vi "RT Init.vi"(6 "Device Outputs FIFO":refnum<k33>, 8 "error in":errorcluster, 11 "Device Ref":T13=18446744073709551615 format="%.0x") -> (0 "error out":errorcluster, 3 "RT Data":T1={"Timekeeper hdl"="", "clkDisc session"=variant, "Compiled Data"={"SyncMod?"=FALSE, "SyncMod"="", "ConnectionSettings"={"Mode"=enum."Generate sample clock", "pxitrig"=FALSE, "pfi0"=FALSE, "pfi1"=FALSE, "pfi2"=FALSE, "External Pin"=enum."PFI0", "Routes"=[]}, "TimeKeeper"="", "ScanOffset(%)"=0.0, "StartDelay(s)"=0, "Time Ref Settings"={"Time Reference"=enum."GPS", "Priority 1"=0, "Priority 2"=0, "IRIG type"=enum."IRIGB AM", "Terminal"="", "PPSSetTime"=FALSE, "Start Time"=timestamp(0 s since 1904-01-01)}, "FIFO Locations"={"BoardTime"=[], "Status"=[]}}, "OutputsData"=[], "OutputsFIFO"=refnum, "Scan Period"=0, "Timekeeper type"=enum."6683", "SyncMod type"=enum."6683", "SyncMod hdl"=""} {"Compiled Data"."Time Ref Settings"."Priority 2" min=0 max=255; "Compiled Data"."Time Ref Settings"."Priority 1" min=0 max=255}, 4 "Name":string)   [LabVIEW 2015, in "Chassis TimeSync Engine.lvlib"]
uses:
  Chassis TimeSync Engine.lvlib
  <vilib>/NI Veristand/Custom Device API/Custom Device Item Ref.ctl
  RT Data Cluster.ctl
  mdevClkDisc.llb/_clkDisc_session.ctl
  Shared/Compiled Data.ctl
  Shared/Connection Settings.ctl
  Shared/Mode.ctl
  Shared/External Pin.ctl
  Shared/Routes.ctl
  Shared/Route.ctl
  Shared/Time Ref Settings.ctl
  Shared/Time Reference.ctl
  Shared/IRIG Type.ctl
  timekeeper type.ctl
  <instrlib>/niSync/niSync.llb/niSync Initialize (Default).vi
  <vilib>/NI Veristand/Custom Device API/Get Item Property (Variant).vi
  Shared/Constants.vi
  <vilib>/NI Veristand/Custom Device API/Custom Device API.lvlib
  Shared/Chassis TimeSync Shared.lvlib
  <vilib>/NI Veristand/Custom Device Tools/Custom Device Utility Library/Custom Device Utility Library.lvlib
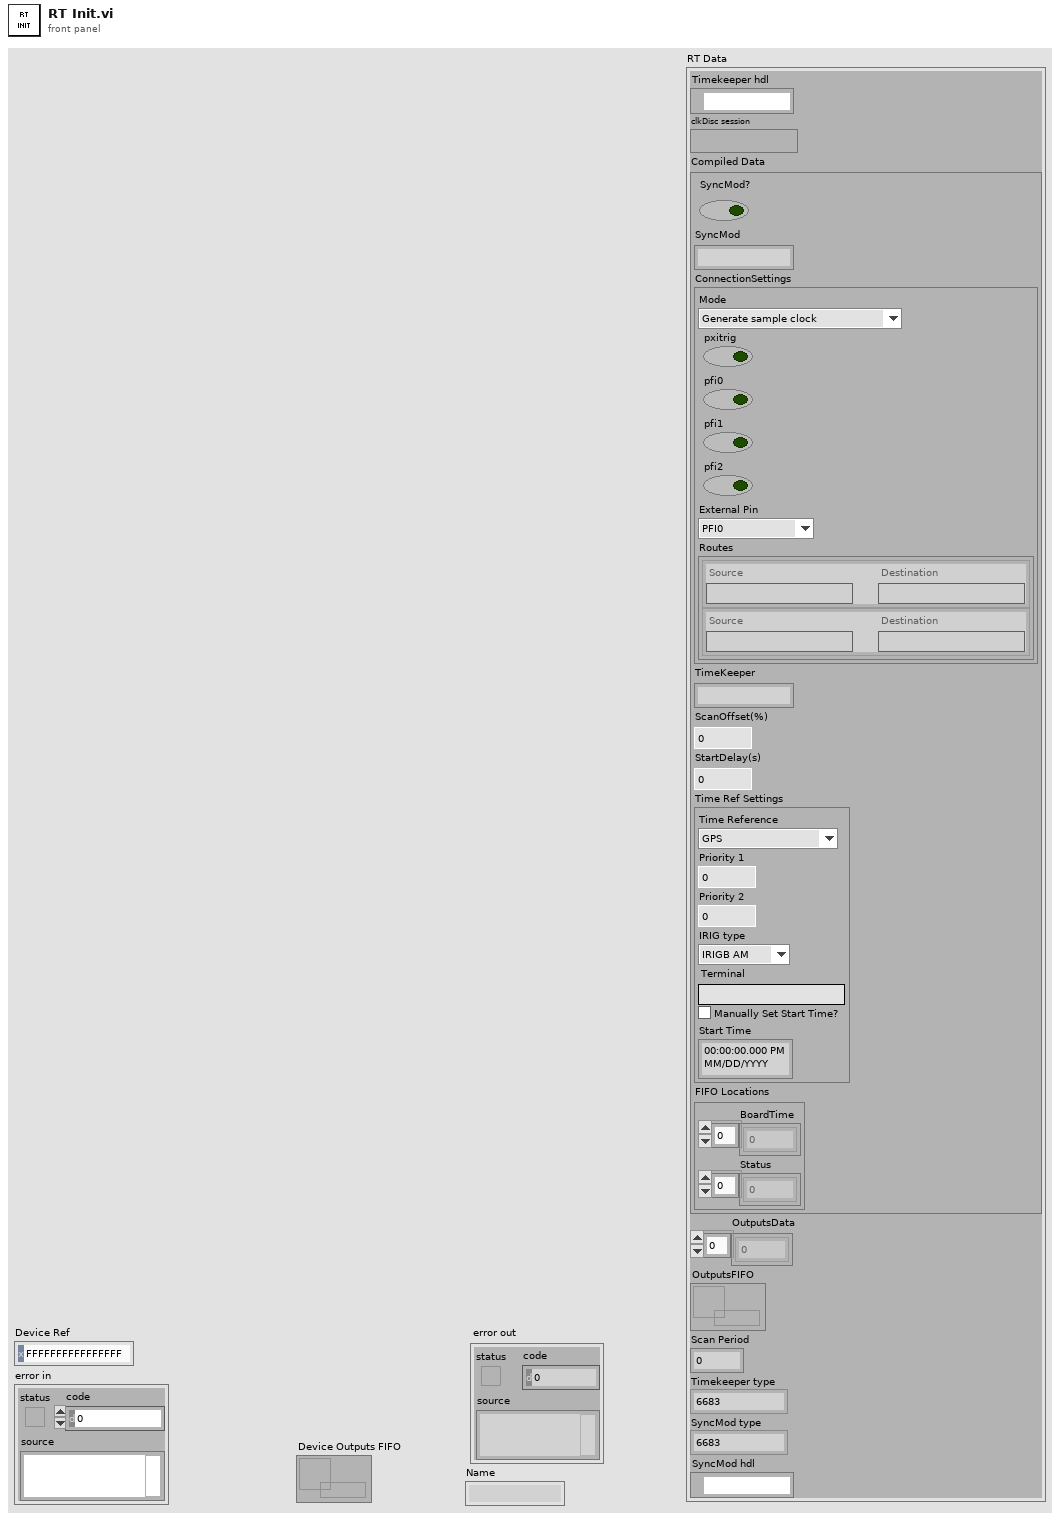
[diagram p1: front panel]
types:
  T1 = typedef "Chassis TimeSync Engine.lvlib/RT Data Cluster.ctl" = cluster{"Timekeeper hdl":refnum<k15>, "clkDisc session":T2, "Compiled Data":T3, "OutputsData":dbl[], "OutputsFIFO":refnum<k33>, "Scan Period":u32, "Timekeeper type":T12, "SyncMod type":T12, "SyncMod hdl":refnum<k15>}
  T2 = typedef "_clkDisc_session.ctl" = variant
  T3 = typedef "Chassis TimeSync Shared.lvlib/Compiled Data.ctl" = cluster{"SyncMod?":bool, "SyncMod":string, "ConnectionSettings":T4, "TimeKeeper":string, "ScanOffset(%)":dbl, "StartDelay(s)":u16, "Time Ref Settings":T9, "FIFO Locations":cluster{"BoardTime":i32[], "Status":i32[]}}
  T4 = typedef "Chassis TimeSync Shared.lvlib/Connection Settings.ctl" = cluster{"Mode":T5, "pxitrig":bool, "pfi0":bool, "pfi1":bool, "pfi2":bool, "External Pin":T6, "Routes":T7}
  T5 = typedef "Chassis TimeSync Shared.lvlib/Mode.ctl" = enum16{"Generate sample clock", "Route sample clock out of chassis", "Route sample clock into chassis", "Custom routes"}
  T6 = typedef "Chassis TimeSync Shared.lvlib/External Pin.ctl" = enum16{"PFI0", "PFI1", "PFI2"}
  T7 = typedef "Chassis TimeSync Shared.lvlib/Routes.ctl" = T8[]
  T8 = typedef "Chassis TimeSync Shared.lvlib/Route.ctl" = cluster{"Source":string, "Destination":string}
  T9 = typedef "Chassis TimeSync Shared.lvlib/Time Ref Settings.ctl" = cluster{"Time Reference":T10, "Priority 1":i32, "Priority 2":i32, "IRIG type":T11, "Terminal":string, "PPSSetTime":bool, "Start Time":timestamp}
  T10 = typedef "Chassis TimeSync Shared.lvlib/Time Reference.ctl" = enum16{"GPS", "IRIG", "PPS", "1588 Ordinary Clock", "PXI Chassis Clock", "Free Running (Internal)"}
  T11 = typedef "Chassis TimeSync Shared.lvlib/IRIG Type.ctl" = enum16{"IRIGB DC", "IRIGB AM"}
  T12 = typedef "Chassis TimeSync Engine.lvlib/timekeeper type.ctl" = enum16{"6683", "6683H", "6682", "6682H", "non-timekeeper", "timekeeper"}
  T13 = typedef "Custom Device API.lvlib/Custom Device Item Ref.ctl" = u64
  T14 = typedef "Custom Device API.lvlib/Custom Device Item Info.ctl" = cluster{"Name":string, "Is Channel":bool, "GUID":string, "Is Waveform":bool}
  T15 = typedef "Custom Device API.lvlib/Custom Device Channel.ctl" = cluster{"Type":T16, "Units":string, "Default Value":dbl, "Faultable":bool, "Scalable":bool}
  T16 = typedef "Custom Device API.lvlib/Custom Device Channel Type.ctl" = enum16{"Input", "Output"}
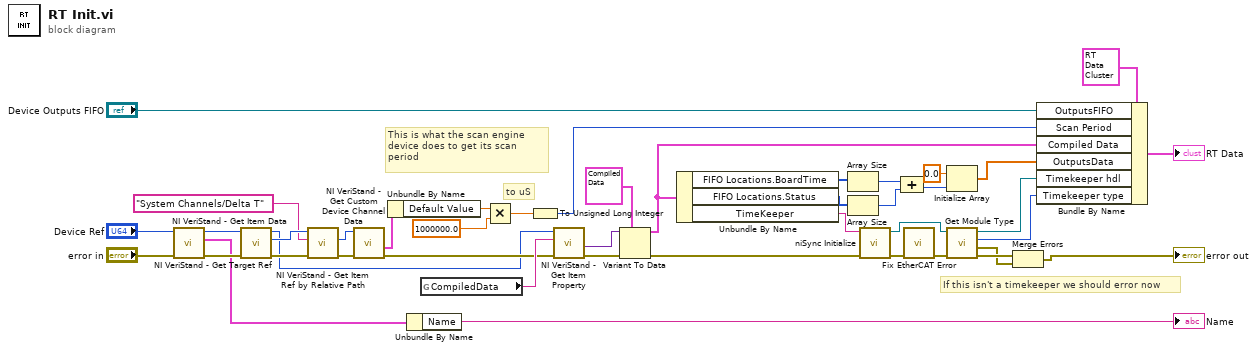
[diagram p0: block diagram]
diagram:
  # "If this isn't a timekeeper we should error now"
  # "This is what the scan engine device does to get its scan period"
  # "to uS"
  n1 = call <vilib>:"NI VeriStand - Get Item Data.vi"("error in (no error)"="error in", "Item Ref in"="Device Ref") -> ("error out"=w13:errorcluster, "Item Info"=w10:T14, "Item Ref out"=w11:T13)  [unwired: 6 in, 1 out]
  n2 = call <vilib>:"NI VeriStand - Get Target Ref.vi"("error in"=w13, "Item Ref in"=w11) -> ("error out"=w21:errorcluster, "Target Ref"=w22:T13, "Item Ref out"=w14:T13)  [unwired: 6 in, 1 out]
  n3 = call <vilib>:"NI VeriStand - Get Item Ref by Relative Path.vi"("error in"=w21, "Relative Item Path"="System Channels/Delta T", "Section Ref in"=w22) -> ("error out"=w18:errorcluster, "Item Ref"=w19:T13)  [unwired: 5 in, 2 out]
  n4 = call <vilib>:"NI VeriStand - Get Custom Device Channel Data.vi"("error in (no error)"=w18, "Channel Ref in"=w19) -> ("error out"=w15:errorcluster, "Channel"=w17:T15)  [unwired: 4 in, 4 out]
  n5 = Unbundle By Name(w17) -> ("Default Value"=w26:dbl)
  n6 = Unbundle By Name(w10) -> ("Name"=→"Name":string)
  n7 = global read "Constants.vi" "CompiledData"() -> (w43:string)
  n8 = Multiply(x=w26, y=1000000.0) -> (x*y=w24:dbl)
  n9 = To Unsigned Long Integer(number=w24) -> (unsigned 32bit integer=w16:u32)
  n10 = call-poly <vilib>:"NI VeriStand - Get Item Property.vi"("error in (no error)"=w15, "Property Name"=w43, "Item Ref in"=w14) -> ("error out"=w42:errorcluster, "Value"=w38:variant)  [unwired: 5 in, 2 out]
  n11 = Variant To Data(error in=w42, type=T3 {"SyncMod?"=FALSE, "SyncMod"="", "ConnectionSettings"={"Mode"=enum."Generate sample clock", "pxitrig"=FALSE, "pfi0"=FALSE, "pfi1"=FALSE, "pfi2"=FALSE, "External Pin"=enum."PFI0", "Routes"=[]}, "TimeKeeper"="", "ScanOffset(%)"=0.0, "StartDelay(s)"=0, "Time Ref Settings"={"Time Reference"=enum."GPS", "Priority 1"=0, "Priority 2"=0, "IRIG type"=enum."IRIGB AM", "Terminal"="", "PPSSetTime"=FALSE, "Start Time"=timestamp(0 s since 1904-01-01)}, "FIFO Locations"={"BoardTime"=[], "Status"=[]}} ("Compiled Data"), Variant=w38) -> (data=w35:T3, error out=w39:errorcluster)
  n12 = Unbundle By Name(w35) -> ("FIFO Locations.BoardTime"=w33:i32[], "FIFO Locations.Status"=w32:i32[], "TimeKeeper"=w36:string)
  n13 = Array Size(array=w33) -> (size(s)=w31:i32)
  n14 = Array Size(array=w32) -> (size(s)=w30:i32)
  n15 = call-poly <instrlib>:"niSync Initialize.vi"("error in (no error)"=w39, "resource name"=w36) -> ("error out"=w2:errorcluster, "instrument handle out"=w8:refnum<k15>)  [unwired: 8 in]
  n16 = Compound Arithmetic op=ADD(w31, w30) -> (w29:i32)
  n17 = call "Fix EtherCAT Error.vi"("error in (no error)"=w2) -> ("error out"=w1:errorcluster)  [unwired: 10 in]
  n18 = Initialize Array(0.0 ("element"), w29) -> (w27:dbl[])
  n19 = call "Get Module Type.vi"("error in (no error)"=w1, "IVI Refnum in"=w8) -> ("error out"=w5:errorcluster, "timekeeper check error out"=w4:errorcluster, "Module type"=w6:T12, "IVI Refnum out"=w7:refnum<k15>)  [unwired: 6 in]
  n20 = Merge Errors(w5, w4) -> (→"error out":errorcluster)
  n21 = Bundle By Name(cluster=T1 {"Timekeeper hdl"="", "clkDisc session"=variant, "Compiled Data"={"SyncMod?"=FALSE, "SyncMod"="", "ConnectionSettings"={"Mode"=enum."Generate sample clock", "pxitrig"=FALSE, "pfi0"=FALSE, "pfi1"=FALSE, "pfi2"=FALSE, "External Pin"=enum."PFI0", "Routes"=[]}, "TimeKeeper"="", "ScanOffset(%)"=0.0, "StartDelay(s)"=0, "Time Ref Settings"={"Time Reference"=enum."GPS", "Priority 1"=0, "Priority 2"=0, "IRIG type"=enum."IRIGB AM", "Terminal"="", "PPSSetTime"=FALSE, "Start Time"=timestamp(0 s since 1904-01-01)}, "FIFO Locations"={"BoardTime"=[], "Status"=[]}}, "OutputsData"=[], "OutputsFIFO"=refnum, "Scan Period"=0, "Timekeeper type"=enum."6683", "SyncMod type"=enum."6683", "SyncMod hdl"=""}, "OutputsFIFO"="Device Outputs FIFO", "Scan Period"=w16, "Compiled Data"=w35, "OutputsData"=w27, "Timekeeper hdl"=w7, "Timekeeper type"=w6) -> (→"RT Data":T1)
